vi "MC5e Squads to Summary Strings.vi"() -> (3 "Squad Strings":string[](array[string]))   [LabVIEW 2020]
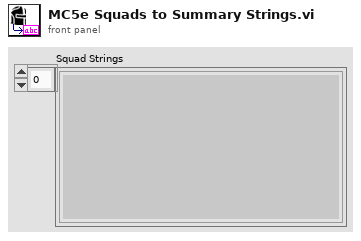
[diagram p1: front panel]
types:
  T1 = typedef "MC5e Squad_Set.ctl" = set{T2}
  T2 = typedef "MC5e Squad_Info.ctl" = cluster{"Squad Name":string, "# Soldiers":u16, "Battle Rating":u16, "Flying":bool, "Mounted":bool, "Speed":u16, "Range":u16, "Morale":i32, "Max Endurance":u16, "Current Endurance":i32, "Size":T3, "Space Taken":u16, "Difficult Terrain":i32[], "CR":u16, "Special / Notes":string}
  T3 = typedef "MC5e Size_Categories.ctl" = enum16{"Tiny", "Small", "Medium", "Large", "Huge", "Gargantuan"}
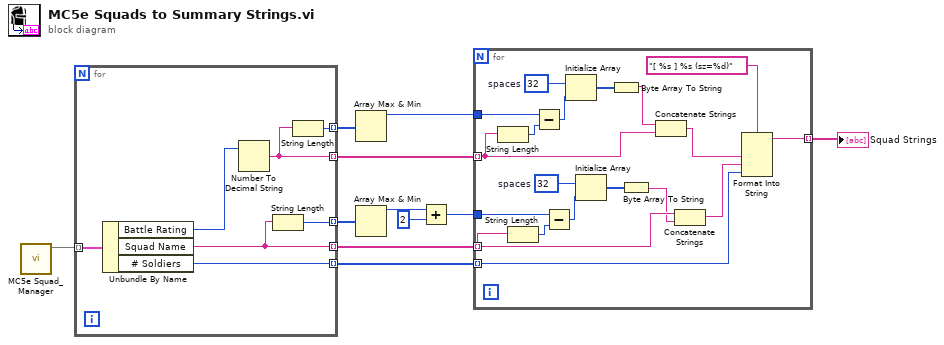
[diagram p0: block diagram]
diagram:
  n1 = call "MC5e Squad_Manager.vi"() -> ("Squad Set"=w1:T1)  [unwired: 8 in, 3 out]
  n2 = for {
    tunnel: w1 -> [w18] mode=indexing
    tunnel: [w16] -> w8 mode=indexing
    tunnel: [w15] -> w11 mode=indexing
    tunnel: [w14] -> w6 mode=indexing
    tunnel: [w13] -> w7 mode=indexing
    tunnel: [w12] -> w2 mode=indexing
    n3 = Unbundle By Name(w18) -> ("Battle Rating"=w17:u16, "Squad Name"=w16:string, "# Soldiers"=w14:u16)
    n4 = Number To Decimal String(number=w17) -> (decimal integer string=w13:string)  [unwired: 1 in]
    n5 = String Length(string=w16) -> (length=w15:i32)
    n6 = String Length(string=w13) -> (length=w12:i32)
  }
  n7 = Array Max & Min(array=w2) -> (max value=w3:i32)  [unwired: 3 out]
  n8 = Array Max & Min(array=w11) -> (max value=w10:i32)  [unwired: 3 out]
  n9 = Add(x=w10, y=2) -> (x+y=w4:i32)
  n10 = for {
    tunnel: w8 -> [w29] mode=indexing
    tunnel: w7 -> [w21] mode=indexing
    tunnel: w6 -> [w36] mode=indexing
    tunnel: [w35] -> w5 mode=indexing
    tunnel: w4 -> [w33]
    tunnel: w3 -> [w22]
    w25 = u8 32  # spaces
    w31 = u8 32  # spaces
    n11 = String Length(string=w21) -> (length=w23:i32)
    n12 = String Length(string=w29) -> (length=w34:i32)
    n13 = Subtract(x=w22, y=w23) -> (x-y=w26:i32)
    n14 = Subtract(x=w33, y=w34) -> (x-y=w30:i32)
    n15 = Initialize Array(w25, w26) -> (w24:u8[])
    n16 = Initialize Array(w31, w30) -> (w32:u8[])
    n17 = Byte Array To String(unsigned byte array=w24) -> (string=w20:string)
    n18 = Byte Array To String(unsigned byte array=w32) -> (string=w28:string)
    n19 = Concatenate Strings(w20, w21) -> (w19:string)
    n20 = Concatenate Strings(w29, w28) -> (w27:string)
    n21 = Format Into String(format string="[ %s ] %s (sz=%d)", w19, w27, w36) -> (resulting string=w35:string)  [unwired: 2 in, 1 out]
  }
  "Squad Strings" <- w5
